vi "Do.vi"(8 "error in (no error)":errorcluster, 10 "Actor in":refnum<class "Actor.lvclass">, 11 "Menu Activation Msg":refnum<class "Menu Activation Msg.lvclass">) -> (0 "error out":errorcluster, 2 "Actor out":refnum<class "Actor.lvclass">)   [LabVIEW 2014, in "HIJ 3 Alignment Cams App.lvlib" / "Menu Activation Msg.lvclass"]
doc: "This VI delivers the message to the actor by calling the appropriate method(s) on the actor."
uses:
  Menu Activation Msg.lvclass
  <vilib>/ActorFramework/Actor/Actor.lvclass
  HIJ 3 Alignment Cams App/HIJ 3 Alignment Cams App.lvclass
  Menu Activation Msg.lvclass/Menu Activation Msg.ctl
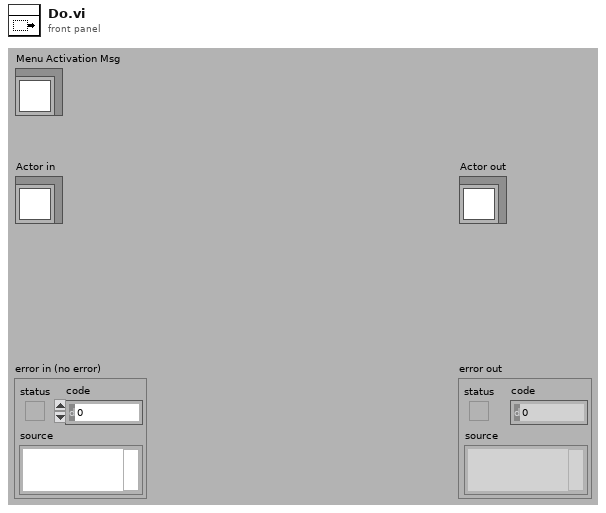
[diagram p1: front panel]
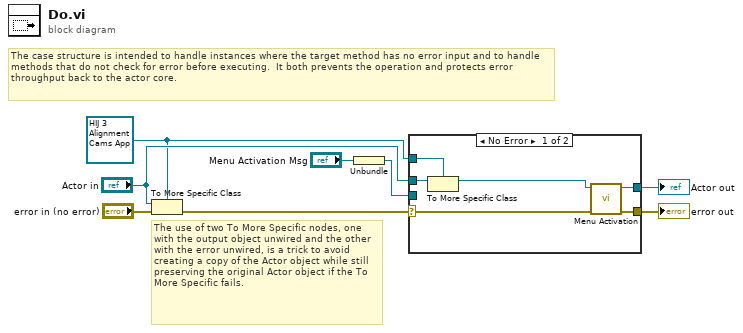
[diagram p0: block diagram]
diagram:
  w2 = refnum<class "HIJ 3 Alignment Cams App.lvclass"> refnum ("Actor in")
  # "The use of two To More Specific nodes, one with the output object unwired and the other with the error unwired, is a trick to avoid creating a copy of the Actor object while still preserving the original Actor object if the To More Specific fails."
  # "The case structure is intended to handle instances where the target method has no error input and to handle methods that do not check for error before executing.  It both prevents the operation and protects error throughput back to the actor core."
  n1 = To More Specific Class(target class=w2, reference="Actor in", error in="error in (no error)") -> (error out=w6:errorcluster)  [unwired: 1 out]
  n2 = Unbundle("Menu Activation Msg") -> (w1:refnum<k9>)
  n3 = case shown="No Error" w6 {
    selector: w6 -> [w12 w16]
    tunnel: [w14 w16] -> w5
    tunnel: [w13 w15] -> w4
    tunnel: "Actor in" -> [w11 w15]
    tunnel: w2 -> [w10 _]
    tunnel: w1 -> [_ _]
    frame No Error {
      n4 = To More Specific Class(target class=w10, reference=w11) -> (specific class reference=w9:refnum<class "HIJ 3 Alignment Cams App.lvclass">)  [unwired: 1 in, 1 out]
      n5 = call "Menu Activation.vi"("error in (no error)"=w12, "HIJ 4 Alignment Cams App in"=w9) -> ("error out"=w14:errorcluster, "HIJ 4 Alignment Cams App out"=w13:refnum<class "HIJ 3 Alignment Cams App.lvclass">)  [unwired: 8 in]
    }
    frame Error {
      # "If type check fails, pass the original object out again."
    }
  }
  "error out" <- w5
  "Actor out" <- w4
